vi "FileNameDialog.vi"(11 "File Name":string) -> (1 "OK?":bool, 3 "String Out":string)   [LabVIEW 2016]
panel:
  in  "Cancel":bool
  in  "OK in":bool caption="OK2"
  # "Enter a file name for your Python code"
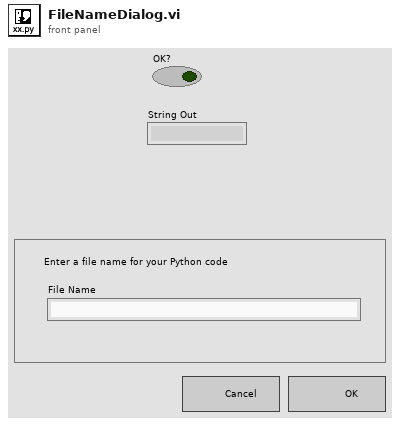
[diagram p1: front panel]
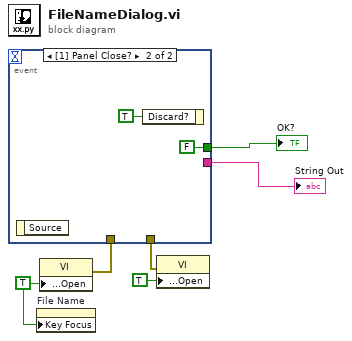
[diagram p0: block diagram]
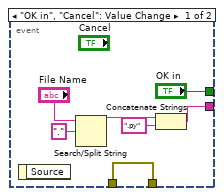
[diagram p2: hidden frame]
diagram:
  w3 = TRUE ("Front Panel Window:Open")
  n1 = property on="File Name" class="Str"("Key Focus"=w3) -> ()  [unwired: 2 in, 2 out]
  n2 = property class="VI"("Front Panel Window:Open"=w3) -> (error out=w6:errorcluster)  [unwired: 2 in, 1 out]
  n3 = event shown="[1] Panel Close?" {
    selector: _ -> [_ _]
    dyn-events: _ -> [_ _]
    timeout: _ -> [_ _]
    tunnel: ["OK in" FALSE ("OK in")] -> w1
    tunnel: [w8 _] -> w2
    tunnel: [w12 _] -> w5
    tunnel: w6 -> [w12 _]
    event "OK in", "Cancel": Value Change {
      n4 = event-data() -> ()  [unwired: 1 in, 1 out]
      n5 = Search/Split String(string="File Name", search string/char (-)=".") -> (substring before match=w10:string)  [unwired: 1 in, 2 out]
      n6 = Concatenate Strings(w10, ".py" ("string")) -> (w8:string)
    }
    event Panel Close? {
      n7 = event-data() -> ()  [unwired: 1 in, 1 out]
      n8 = event-data("Discard?"=TRUE) -> ()  [unwired: 1 in, 1 out]
    }
  }
  "String Out" <- w2
  "OK?" <- w1
  n9 = property class="VI"(error in=w5, "Front Panel Window:Open"=TRUE) -> ()  [unwired: 1 in, 2 out]
